vi "open MB.vi"(4 "Port (502)":u16=502, 6 "IP Address":string="localhost", 7 "MODE":u16(ring) items=["Modbus RTU", "Modbus TCP"], 8 "error in (no error)":errorcluster caption="错误输入（无错误）", 9 "Serial Config":T1={"baud rate (bps)"=19200, "stop bits"=10, "parity"=0, "flow control"=0, "timeout"=1000, "retries"=1} {"stop bits" items=["1.0"=10, "1.5"=15, "2.0"=20]; "parity" items=["None", "Odd", "Even", "Mark", "Space"]; "flow control" items=["None", "XON/XOFF", "RTS/CTS", "XON/XOFF & RTS/CTS", "DTR/DSR", "XON/XOFF & DTR/DSR"]}, 10 "Slave ID":u8=1, 11 "VISA资源名称":refnum<visa-resource-name>) -> (0 "error out":errorcluster caption="错误输出", 3 "MB session out":refnum<class "MB_Master.lvclass">)   [LabVIEW 2016, in "斯坦道多参数.lvlib"]
uses:
  <vilib>/Plasmionique/MB Master/MB_Master/MB_Master.lvclass
  <vilib>/Plasmionique/MB Master/MB_Master_Serial/MB_Master_Serial.lvclass
  D:/Program Files (x86)/National Instruments/LabVIEW 2016/vi.lib/Plasmionique/MB Master/MB_Master/MB_Master.lvclass
  <vilib>/Plasmionique/MB Master/MB_Master_TCP/MB_Master_TCP.lvclass
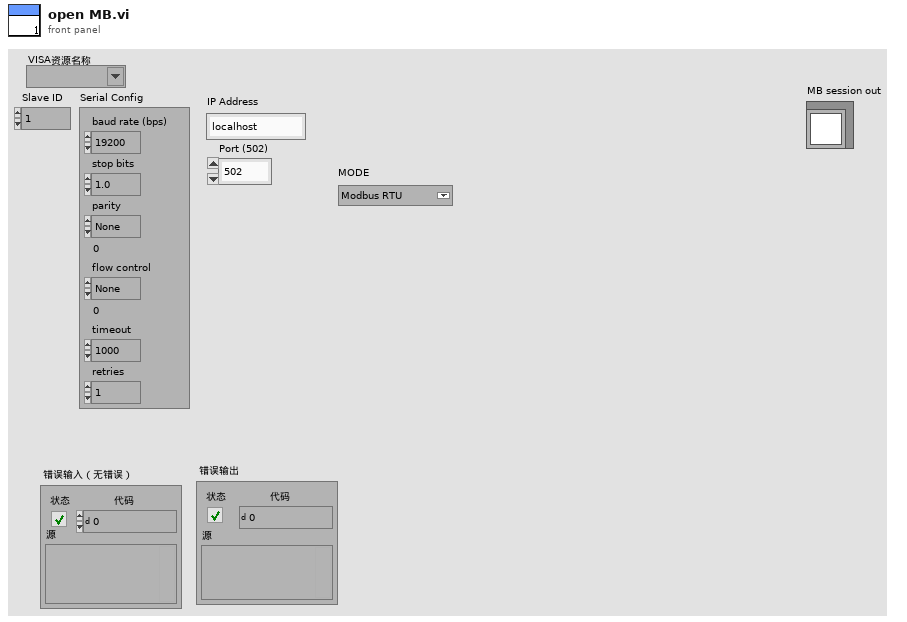
[diagram p1: front panel]
types:
  T1 = cluster{"baud rate (bps)":u32, "stop bits":u16, "parity":u16, "flow control":u16, "timeout":u32, "retries":i32}
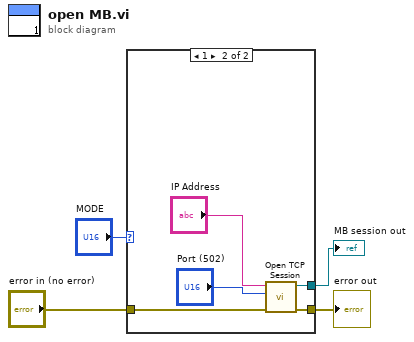
[diagram p0: block diagram]
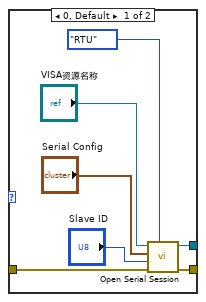
[diagram p2: hidden frame]
diagram:
  n1 = case shown="1" "MODE" {
    tunnel: "error in (no error)" -> [w7 w16]
    tunnel: [w6 w15] -> w3
    tunnel: [w5 w14] -> w1
    frame 0, Default {
      n2 = call <vilib>:"Open Serial Session.vi"("Mode (RTU)"=enum16{"RTU", "ASCII"}."RTU", "Error in"=w7, "Slave ID"="Slave ID", "Serial Config"="Serial Config", "VISA Resource"="VISA资源名称") -> ("Error out"=w6:errorcluster, "MB_Serial session"=w5:refnum<class "MB_Master_Serial.lvclass">)  [unwired: 5 in]
    }
    frame 1 {
      n3 = call <vilib>:"Open TCP Session.vi"("error in (no error)"=w16, "Port (502)"="Port (502)", "IP Address"="IP Address") -> ("error out"=w15:errorcluster, "MB_TCP session"=w14:refnum<class "MB_Master_TCP.lvclass">)  [unwired: 7 in]
    }
  }
  "error out" <- w3
  "MB session out" <- w1
